vi "SetAzCamToolParameter.vi"(1 "Value":string, 2 "Parameter":string) -> (0 "Error":bool)   [LabVIEW 2014]
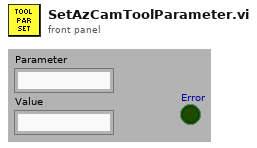
[diagram p1: front panel]
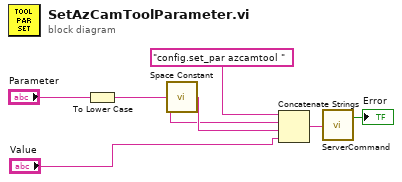
[diagram p0: block diagram]
diagram:
  n1 = To Lower Case(string="Parameter") -> (all lower case string=w2:string)
  n2 = call <vilib>:"Space Constant.vi"() -> ("String"=w4:string)
  n3 = Concatenate Strings("config.set_par azcamtool " ("Attribute"), w2, w4, "Value") -> (w7:string)
  n4 = call "ServerCommand.vi"("Command"=w7) -> ("Error"=→"Error":bool)  [unwired: 1 out]
